vi "Evaluate Part 2.vi"() -> ()   [LabVIEW 2020]
uses:
  Descrambler/Descrambler.lvclass
  Words to Numbers Converter/Words to Numbers Converter.lvclass
panel:
  out "string array":string[](array[string])
  out "Numbers":i32[](array[numeric])
  out "sum":i32=142
  in  "Input":string="1abc2\npqr3stu8vwx\na1b2c3d4e5f\ntreb7uchet"
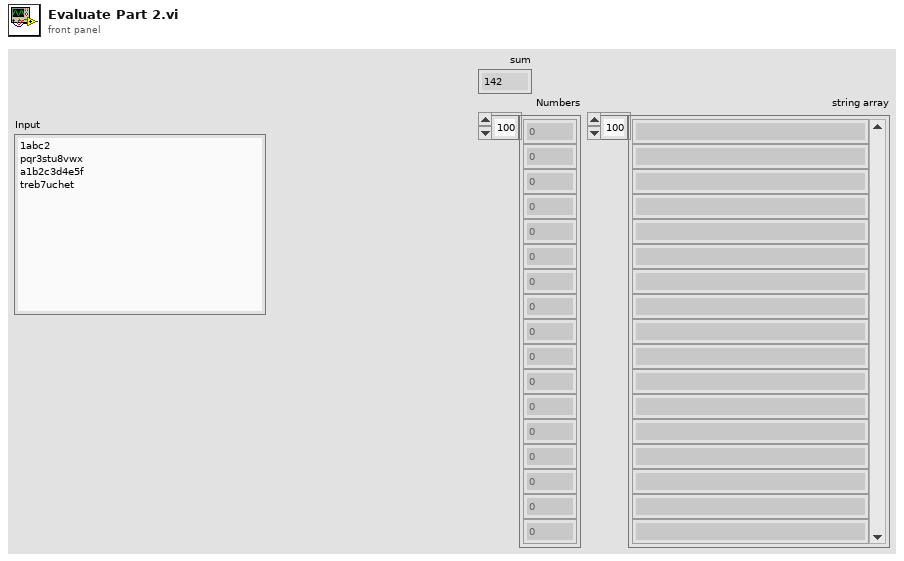
[diagram p1: front panel]
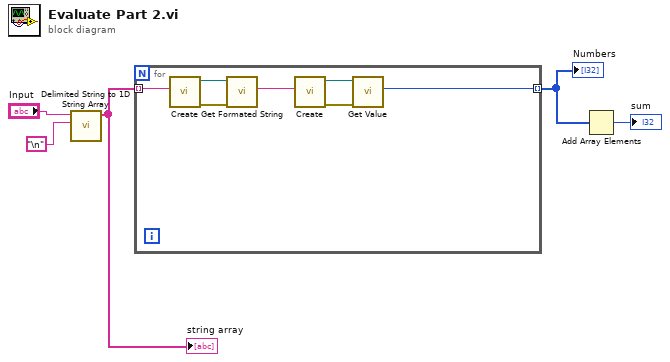
[diagram p0: block diagram]
diagram:
  n1 = call <vilib>:"Delimited String to 1D String Array.vi"("delimiter"="\n", "delimited string"="Input") -> ("string array"=w3:string[])  [unwired: 9 in]
  "string array" <- w3
  n2 = for {
    tunnel: w3 -> [w6] mode=indexing
    tunnel: [w10] -> w2 mode=indexing
    n3 = call "Create.vi"("String"=w6) -> ("error out"=w8:errorcluster, "Words to Numbers Converter"=w9:refnum<class "Words to Numbers Converter.lvclass">)  [unwired: 9 in]
    n4 = call "Get Formated String.vi"("error in (no error)"=w8, "Words to Numbers Converter in"=w9) -> ("String"=w7:string)  [unwired: 7 in, 2 out]
    n5 = call "Create.vi"("String"=w7) -> ("error out"=w11:errorcluster, "Descrambler"=w12:refnum<class "Descrambler.lvclass">)  [unwired: 9 in]
    n6 = call "Get Value.vi"("error in (no error)"=w11, "Descrambler in"=w12) -> ("Value"=w10:i32)  [unwired: 7 in, 2 out]
  }
  "Numbers" <- w2
  n7 = Add Array Elements(numeric array=w2) -> (sum=→"sum":i32)
